vi "MM6Archiver.ProcCases.vi"(0 "i ref in":refnum<vi>, 1 "selector":string, 2 "Data":T1, 3 "call cluster":T2={"Object"="", "Selector"="", "CallType"=enum."synchronous", "Async Object"="", "Async Selector"="", "Data Descriptor"="", "Data"=[], "Error #"=0, "Expire"=0}, 5 "error in (no error)":errorcluster) -> (14 "i ref out":refnum<vi>, 17 "answer cluster":T2={"Object"="", "Selector"="", "CallType"=enum."synchronous", "Async Object"="", "Async Selector"="", "Data Descriptor"="", "Data"=[], "Error #"=0, "Expire"=0}, 19 "error out":errorcluster)   [LabVIEW 2014, in "MM6Archiver.lvlib"]
doc: "This method is called by a process from within the default case in the event loop. The methods of a class that are linked to events will be called from THIS method. Add your code here."
uses:
  MM6Archiver.lvlib
  CSCore/CSSystem/CoreDefs/CoreDefs.call_type.ctl
  CSCore/BaseProcess/BaseProcess.descriptor string definition.ctl
  CSCore/CSSystem/CoreDefs/CoreDefs.rawDataType.ctl
  CSCore/CSSystem/CoreLib/CoreLib.string 2 byte array.vi
  CSCore/BaseProcess/BaseProcess.lvlib
  CSCore/CSSystem/CoreLib/CoreLib.lvlib
  CSData/DiscArchiver/DiscArchiver.lvlib
  CSCore/CAEObj/CAEObj.lvlib
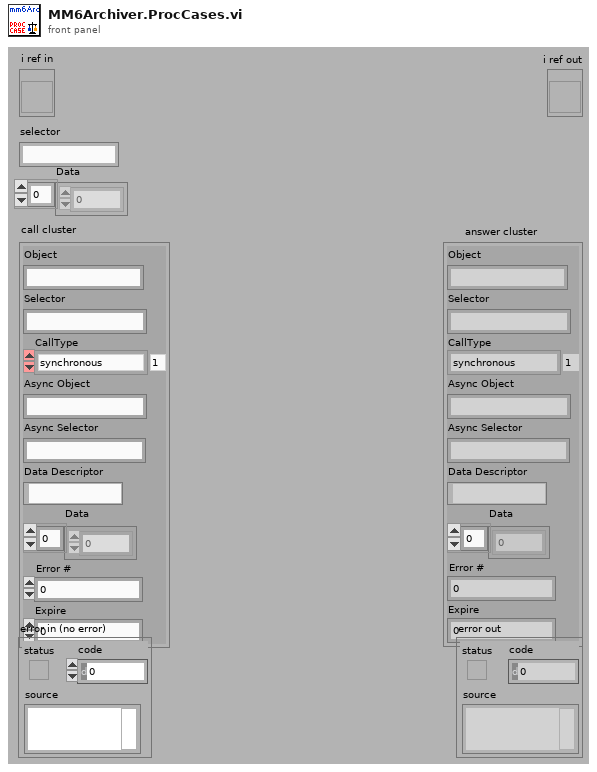
[diagram p1: front panel]
types:
  T1 = typedef "CoreDefs.rawDataType.ctl" = i8[]
  T2 = typedef "CoreDefs.call_type.ctl" = cluster{"Object":string, "Selector":string, "CallType":enum16{"simple", "synchronous", "asynchronous"}, "Async Object":string, "Async Selector":string, "Data Descriptor":T3, "Data":T1, "Error #":i32, "Expire":u32}
  T3 = typedef "BaseProcess.lvlib/BaseProcess.descriptor string definition.ctl" = string
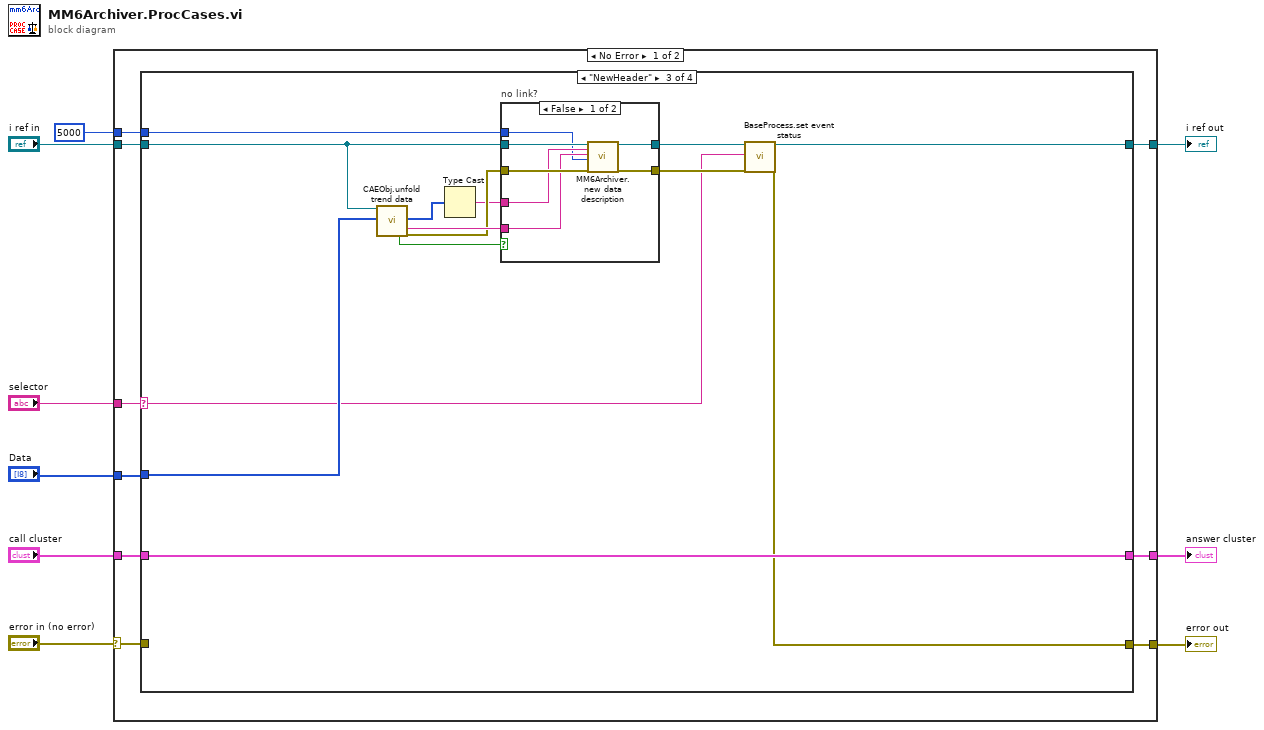
[diagram p0: block diagram]
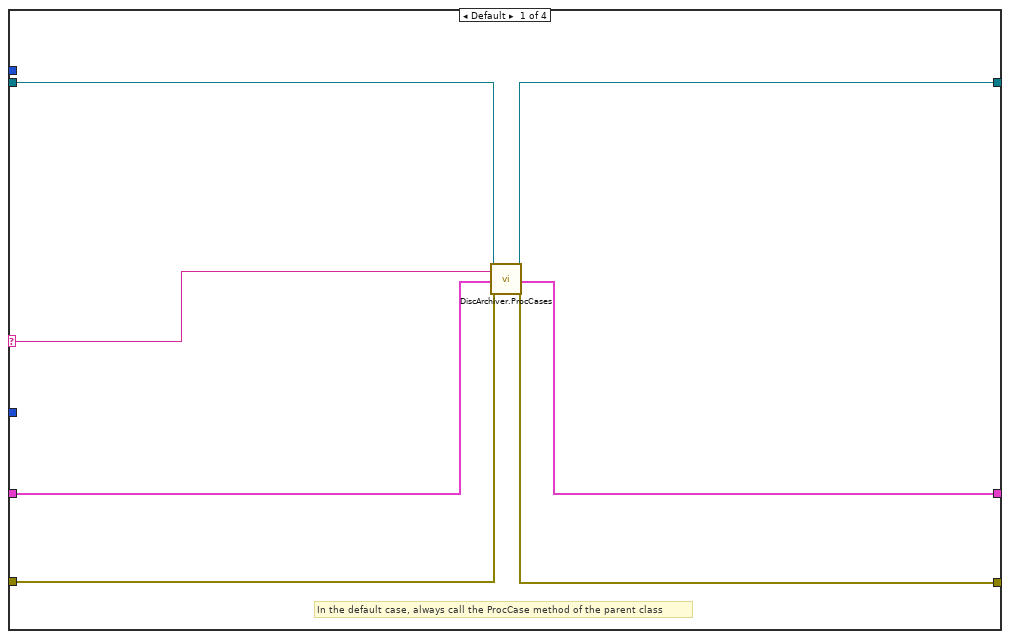
[diagram p2: hidden frame]
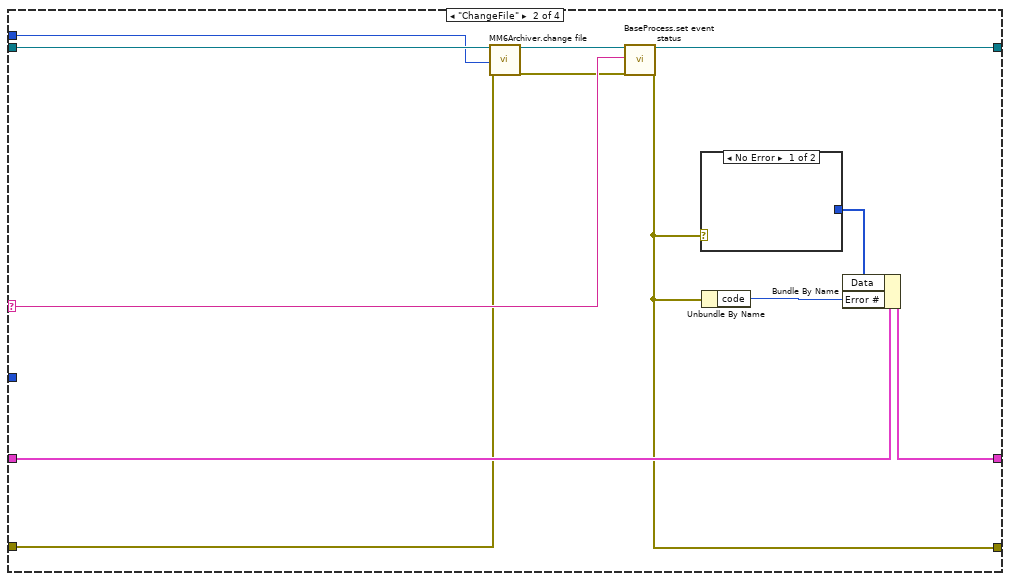
[diagram p3: hidden frame]
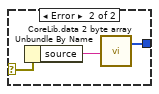
[diagram p4: hidden frame]
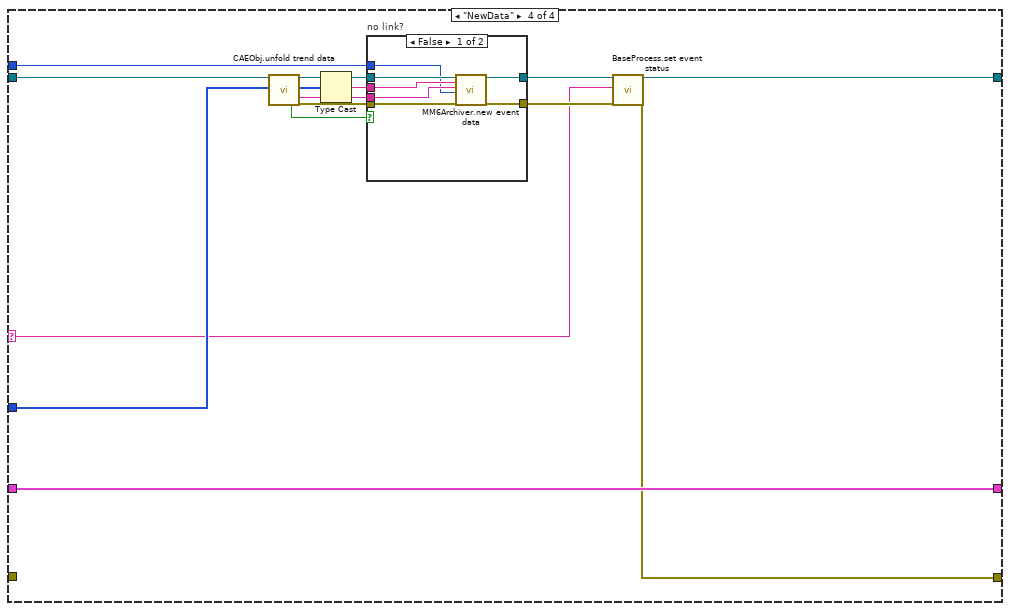
[diagram p6: hidden frame]
diagram:
  n1 = case shown="No Error" "error in (no error)" {
    selector: "error in (no error)" -> [w11 w88]
    tunnel: "selector" -> [w18 _]
    tunnel: [w17 w89] -> w8
    tunnel: "Data" -> [w16 _]
    tunnel: "call cluster" -> [w15 w89]
    tunnel: "i ref in" -> [w14 w90]
    tunnel: [w13 w90] -> w4
    tunnel: [w12 w88] -> w3
    tunnel: 5000 -> [w10 _]
    frame No Error {
      n2 = case shown="\"NewHeader\"" w18 {
        selector: w18 -> [w20 w32 w45 w67]
        tunnel: w16 -> [_ _ w47 w69]
        tunnel: w14 -> [w19 w30 w41 w70]
        tunnel: [w25 w31 w44 w66] -> w13
        tunnel: w15 -> [w21 w36 w43 w65]
        tunnel: [w22 w35 w43 w65] -> w17
        tunnel: w11 -> [w24 w28 _ _]
        tunnel: [w23 w33 w42 w64] -> w12
        tunnel: w10 -> [_ w26 w46 w68]
        frame Default {
          # "In the default case, always call the ProcCase method of the parent class"
          n3 = call "DiscArchiver.ProcCases.vi"("i ref in"=w19, "selector"=w20, "call cluster"=w21, "error in (no error)"=w24) -> ("i ref out"=w25:refnum<vi>, "answer cluster"=w22:T2, "error out"=w23:errorcluster)  [unwired: 13 in]
        }
        frame "ChangeFile" {
          n4 = call "MM6Archiver.change file.vi"("i ref in"=w30, "ms timeout (10000)"=w26, "error in (no error)"=w28) -> ("i ref out"=w29:refnum<vi>, "error out"=w27:errorcluster)  [unwired: 14 in, 1 out]
          n5 = call "BaseProcess.set event status.vi"("i ref in"=w29, "EventStatus"=w32, "error in (no error)"=w27) -> ("i ref out"=w31:refnum<vi>, "error out"=w33:errorcluster)  [unwired: 14 in, 1 out]
          n6 = case shown="No Error" w33 {
            selector: w33 -> [_ w40]
            tunnel: [_ w39] -> w34
            frame No Error {
            }
            frame Error {
              n7 = Unbundle By Name(w40) -> ("source"=w38:string)
              n8 = call-poly "CoreLib.data 2 byte array.vi"("string"=w38) -> ("byteArray out"=w39:T1)  [unwired: 18 in]
            }
          }
          n9 = Unbundle By Name(w33) -> ("code"=w37:i32)
          n10 = Bundle By Name(cluster=w36, "Data"=w34, "Error #"=w37) -> (w35:T2)
        }
        frame "NewHeader" {
          n11 = call "CAEObj.unfold trend data.vi"("i ref in"=w41, "raw trend data"=w47) -> ("no link"=w48:bool, "data"=w49:i8[], "typeDescriptor"=w52:string, "error out"=w51:errorcluster)  [unwired: 9 in, 5 out]
          n12 = Type Cast(x=w49) -> (*(type *) &x=w50:string)  [unwired: 1 in]
          n13 = case "no link?" shown="False" w48 {
            tunnel: [w57 w63] -> w53
            tunnel: w41 -> [w60 w63]
            tunnel: w50 -> [w59 _]
            tunnel: w51 -> [w61 w62]
            tunnel: w52 -> [w58 _]
            tunnel: [w56 w62] -> w54
            tunnel: w46 -> [w55 _]
            frame False {
              n14 = call "MM6Archiver.new data description.vi"("i ref"=w60, "dataDescription"=w59, "descriptor"=w58, "ms timeout (10000)"=w55, "error in (no error)"=w61) -> ("i ref out"=w57:refnum<vi>, "error out"=w56:errorcluster)  [unwired: 12 in, 1 out]
            }
            frame True {
            }
          }
          n15 = call "BaseProcess.set event status.vi"("i ref in"=w53, "EventStatus"=w45, "error in (no error)"=w54) -> ("i ref out"=w44:refnum<vi>, "error out"=w42:errorcluster)  [unwired: 14 in, 1 out]
        }
        frame "NewData" {
          n16 = call "CAEObj.unfold trend data.vi"("i ref in"=w70, "raw trend data"=w69) -> ("no link"=w71:bool, "i ref out"=w74:refnum<vi>, "data"=w72:i8[], "typeDescriptor"=w76:string, "error out"=w75:errorcluster)  [unwired: 9 in, 4 out]
          n17 = Type Cast(x=w72) -> (*(type *) &x=w73:string)  [unwired: 1 in]
          n18 = case "no link?" shown="False" w71 {
            tunnel: [w81 w87] -> w77
            tunnel: w74 -> [w84 w87]
            tunnel: w73 -> [w83 _]
            tunnel: w75 -> [w85 w86]
            tunnel: w76 -> [w82 _]
            tunnel: [w80 w86] -> w78
            tunnel: w68 -> [w79 _]
            frame False {
              n19 = call "MM6Archiver.new event data.vi"("i ref"=w84, "eventData"=w83, "descriptor"=w82, "ms timeout (10000)"=w79, "error in (no error)"=w85) -> ("i ref out"=w81:refnum<vi>, "error out"=w80:errorcluster)  [unwired: 12 in, 1 out]
            }
            frame True {
            }
          }
          n20 = call "BaseProcess.set event status.vi"("i ref in"=w77, "EventStatus"=w67, "error in (no error)"=w78) -> ("i ref out"=w66:refnum<vi>, "error out"=w64:errorcluster)  [unwired: 14 in, 1 out]
        }
      }
    }
    frame Error {
    }
  }
  "answer cluster" <- w8
  "i ref out" <- w4
  "error out" <- w3
